vi "Read and Buffer LLP Packets From Host.vi"(0 "channel configuration":T9, 1 "reset":bool, 2 "resources":T1, 12 "ready for output":bool) -> (4 "tagged llp packet":T10, 6 "end of data":bool, 8 "dram status":T19, 10 "output valid":bool)   [LabVIEW 2020, in "GettingStarted_Gen_148X_FPGA.lvlib"]
uses:
  GettingStarted_Gen_148X_FPGA.lvlib
  Common/Types/DRAM Status.ctl
  <instrlib>/FlexRIO/CSI-2/v2/FPGA/Types/Tagged LLP Packet.ctl
  <instrlib>/FlexRIO/CSI-2/v2/FPGA/Types/FPGA LLP Packet Tag.ctl
  <instrlib>/FlexRIO/CSI-2/v2/FPGA/Types/FPGA LLP Packet Timestamp.ctl
  <instrlib>/FlexRIO/CSI-2/v2/FPGA/Types/Timestamp ID.ctl
  <instrlib>/FlexRIO/CSI-2/v2/FPGA/Types/FPGA LLP Packet Size.ctl
  <instrlib>/FlexRIO/CSI-2/v2/FPGA/Types/LLP Packet.ctl
  <instrlib>/FlexRIO/CSI-2/v2/FPGA/Types/LLP Packet Header.ctl
  <instrlib>/FlexRIO/CSI-2/v2/FPGA/Types/LLP Packet Payload.ctl
  <instrlib>/FlexRIO/CSI-2/v2/FPGA/Types/LLP Packet Footer.ctl
  Types/Serial Output Channel Datapath Configuration.ctl
  Types/Serial Output DRAM Resources.ctl
  <instrlib>/_niInstr/Memory/v1/FPGA/DRAM/niInstr Memory DRAM v1 FPGA.lvclass
  <instrlib>/FlexRIO/CSI-2/v2/FPGA/DRAM Manager/Private/DRAM Manager.ctl
  <instrlib>/FlexRIO/CSI-2/v2/FPGA/DRAM Manager/Private/Common/DRAM Manager Registers.ctl
  <instrlib>/FlexRIO/CSI-2/v2/FPGA/DRAM Manager/Private/Common/Handshake Registers.ctl
  <instrlib>/FlexRIO/CSI-2/v2/FPGA/DRAM Manager/Private/Common/DRAM Manager FIFOs.ctl
  <instrlib>/FlexRIO/CSI-2/v2/FPGA/DRAM Manager/Private/Common/Write Data FIFO Ref.ctl
  <instrlib>/FlexRIO/CSI-2/v2/FPGA/DRAM Manager/Private/Common/Read Request Metadata FIFO Ref.ctl
  <instrlib>/FlexRIO/CSI-2/v2/FPGA/DRAM Manager/Private/Common/Read Data FIFO Ref.ctl
  Common/GettingStarted_Common_148X_FPGA.lvlib
  <instrlib>/_niInstr/Basic Elements/v1/FPGA/niInstr Basic Elements v1 FPGA.lvlib
  <instrlib>/FlexRIO/CSI-2/v2/FPGA/NI CSI-2 API FPGA v2.lvlib
  <instrlib>/FlexRIO/CSI-2/v2/FPGA/DRAM Manager/DRAM Manager v2.lvlib
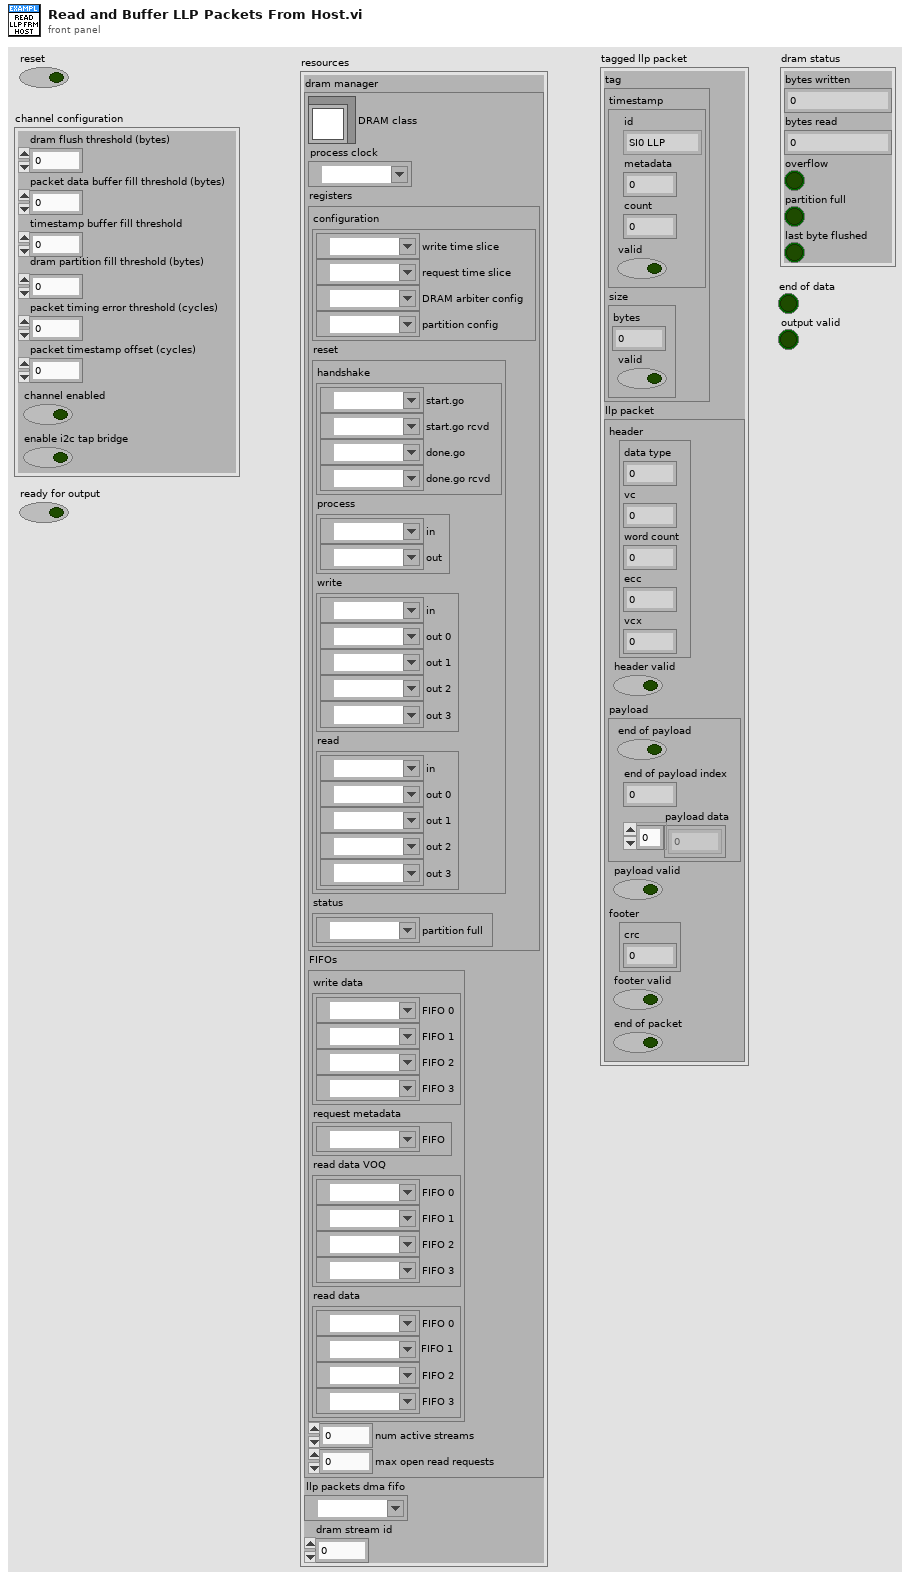
[diagram p1: front panel]
types:
  T1 = typedef "GettingStarted_Gen_148X_FPGA.lvlib/Serial Output DRAM Resources.ctl" = cluster{"dram manager":T2, "llp packets dma fifo":refnum<k21>, "dram stream id":fxp<+,2,2>}
  T2 = typedef "DRAM Manager v2.lvlib/DRAM Manager.ctl" = cluster{"DRAM class":refnum<class "niInstr Memory DRAM v1 FPGA.lvclass">, "process clock":refnum<k21>, "registers":T3, "FIFOs":T5, "num active streams":fxp<+,3,3>, "max open read requests":u16}
  T3 = typedef "DRAM Manager v2.lvlib/DRAM Manager Registers.ctl" = cluster{"configuration":cluster{"write time slice":refnum<k21>, "request time slice":refnum<k21>, "DRAM arbiter config":refnum<k21>, "partition config":refnum<k21>}, "reset":cluster{"handshake":T4, "process":cluster{"in":refnum<k21>, "out":refnum<k21>}, "write":cluster{"in":refnum<k21>, "out 0":refnum<k21>, "out 1":refnum<k21>, "out 2":refnum<k21>, "out 3":refnum<k21>}, "read":cluster{"in":refnum<k21>, "out 0":refnum<k21>, "out 1":refnum<k21>, "out 2":refnum<k21>, "out 3":refnum<k21>}}, "status":cluster{"partition full":refnum<k21>}}
  T4 = typedef "DRAM Manager v2.lvlib/Handshake Registers.ctl" = cluster{"start.go":refnum<k21>, "start.go rcvd":refnum<k21>, "done.go":refnum<k21>, "done.go rcvd":refnum<k21>}
  T5 = typedef "DRAM Manager v2.lvlib/DRAM Manager FIFOs.ctl" = cluster{"write data":cluster{"FIFO 0":T6, "FIFO 1":T6, "FIFO 2":T6, "FIFO 3":T6}, "request metadata":cluster{"FIFO":T7}, "read data VOQ":cluster{"FIFO 0":T8, "FIFO 1":T8, "FIFO 2":T8, "FIFO 3":T8}, "read data":cluster{"FIFO 0":T8, "FIFO 1":T8, "FIFO 2":T8, "FIFO 3":T8}}
  T6 = typedef "DRAM Manager v2.lvlib/Write Data FIFO Ref.ctl" = refnum<k21>
  T7 = typedef "DRAM Manager v2.lvlib/Read Request Metadata FIFO Ref.ctl" = refnum<k21>
  T8 = typedef "DRAM Manager v2.lvlib/Read Data FIFO Ref.ctl" = refnum<k21>
  T9 = typedef "GettingStarted_Gen_148X_FPGA.lvlib/Serial Output Channel Datapath Configuration.ctl" = cluster{"dram flush threshold (bytes)":u64, "packet data buffer fill threshold (bytes)":u64, "timestamp buffer fill threshold":u32, "packet timing error threshold (cycles)":u64, "channel enabled":bool, "dram partition fill threshold (bytes)":u64, "enable i2c tap bridge":bool, "packet timestamp offset (cycles)":i64}
  T10 = typedef "NI CSI-2 API FPGA v2.lvlib/Tagged LLP Packet.ctl" = cluster{"tag":T11, "llp packet":T15}
  T11 = typedef "NI CSI-2 API FPGA v2.lvlib/FPGA LLP Packet Tag.ctl" = cluster{"timestamp":T12, "size":T14}
  T12 = typedef "NI CSI-2 API FPGA v2.lvlib/FPGA LLP Packet Timestamp.ctl" = cluster{"valid":bool, "count":fxp<+,50,50>, "id":T13, "metadata":u8}
  T13 = typedef "NI CSI-2 API FPGA v2.lvlib/Timestamp ID.ctl" = enum8{"SI0 LLP", "SI1 LLP", "SI2 LLP", "SI3 LLP", "SI4 LLP", "SI5 LLP", "SI6 LLP", "SI7 LLP", "SO0 LLP", "SO1 LLP", "SO2 LLP", "SO3 LLP", "SO4 LLP", "SO5 LLP", "SO6 LLP", "SO7 LLP", "Ser0 GPIO Bank", "Ser1 GPIO Bank", "Ser2 GPIO Bank", "Ser3 GPIO Bank", "Ser4 GPIO Bank", "Ser5 GPIO Bank", "Ser6 GPIO Bank", "Ser7 GPIO Bank", "Des0 GPIO Bank", "Des1 GPIO Bank", "Des2 GPIO Bank", "Des3 GPIO Bank", "Des4 GPIO Bank", "Des5 GPIO Bank", "Des6 GPIO Bank", "Des7 GPIO Bank", "User0", "User1", "User2", "User3", "User4", "User5", "User6", "User7", "User8", "User9", "User10", "User11", "User12", "User13", "User14", "User15", "User16", "User17", "User18", "User19", "User20", "User21", "User22", "User23", "User24", "User25", "User26", "User27", "User28", "User29", "User30", "User31"}
  T14 = typedef "NI CSI-2 API FPGA v2.lvlib/FPGA LLP Packet Size.ctl" = cluster{"bytes":fxp<+,17,17>, "valid":bool}
  T15 = typedef "NI CSI-2 API FPGA v2.lvlib/LLP Packet.ctl" = cluster{"header":T16, "header valid":bool, "payload":T17, "payload valid":bool, "footer":T18, "footer valid":bool, "end of packet":bool}
  T16 = typedef "NI CSI-2 API FPGA v2.lvlib/LLP Packet Header.ctl" = cluster{"word count":u16, "ecc":fxp<+,6,6>, "vcx":fxp<+,2,2>, "data type":fxp<+,6,6>, "vc":fxp<+,2,2>}
  T17 = typedef "NI CSI-2 API FPGA v2.lvlib/LLP Packet Payload.ctl" = cluster{"end of payload":bool, "end of payload index":fxp<+,3,3>, "payload data":u8[]}
  T18 = typedef "NI CSI-2 API FPGA v2.lvlib/LLP Packet Footer.ctl" = cluster{"crc":u16}
  T19 = typedef "GettingStarted_Common_148X_FPGA.lvlib/DRAM Status.ctl" = cluster{"bytes written":u64, "bytes read":u64, "overflow":bool, "partition full":bool, "last byte flushed":bool}
  T20 = typedef "niInstr Memory v1 FPGA.lvclass/U256.ctl" = bool[]
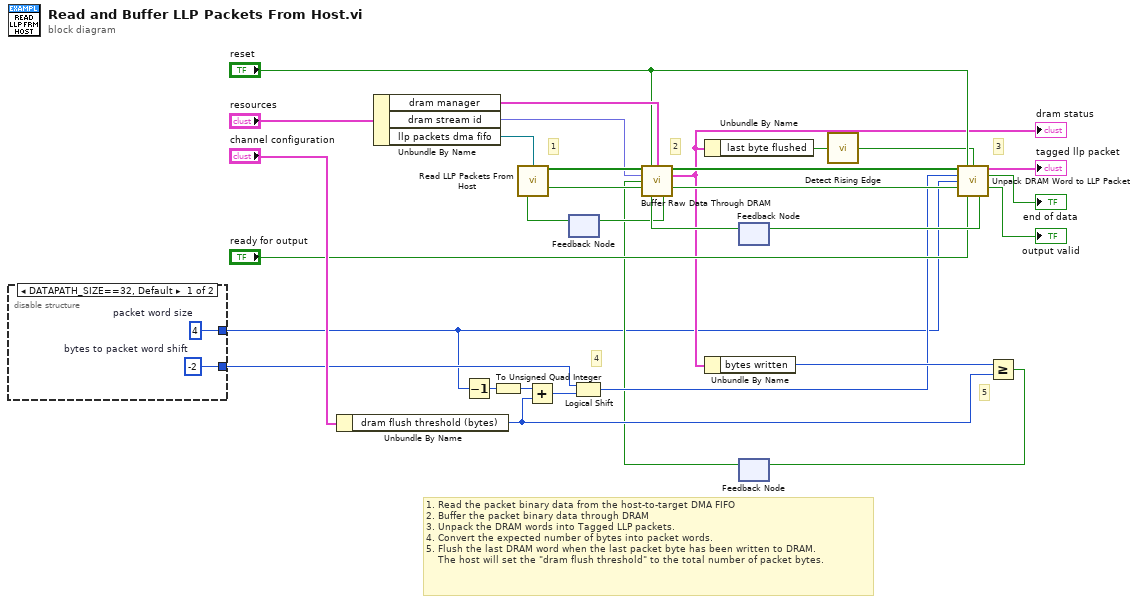
[diagram p0: block diagram]
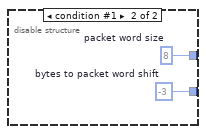
[diagram p2: hidden frame]
diagram:
  # "3"
  # "1. Read the packet binary data from the host-to-target DMA FIFO\n2. Buffer the packet binary data through DRAM\n3. Unpack the DRAM words into Tagged LLP packets.\n4. Convert the expected number of bytes into packet words. \n5. Flush the last DRAM word when the last packet byte has been written to DRAM.\n    The host will set the \"dram flush threshold\" to the total number of packet bytes."
  # "5"
  # "4"
  # "2"
  # "1"
  n1 = disable-structure shown="DATAPATH_SIZE==32, Default" {
    disable-tunnel: [w33 w35] -> w3
    disable-tunnel: [w32 w34] -> w4
    frame condition #0 (active) {
      w32 = i16 -2  # bytes to packet word shift
      w33 = u16 4  # packet word size
    }
    frame condition #1 {
      w34 = i16 -3  # bytes to packet word shift
      w35 = u16 8  # packet word size
    }
  }
  n2 = Unbundle By Name("channel configuration") -> ("dram flush threshold (bytes)"=w13:u64)
  n3 = Unbundle By Name("resources") -> ("dram manager"=w22:T2, "dram stream id"=w21:fxp<+,2,2>, "llp packets dma fifo"=w31:refnum<k21>)
  n4 = Decrement(x=w3) -> (x-1=w2:u16)
  n5 = To Unsigned Quad Integer(1:w2) -> (0:w1:u64)
  n6 = Add(x=w1, y=w13) -> (x+y=w23:u64)
  n7 = feedback #1() -> (w28:bool)  [unwired: 1 in]
  n8 = call "Read LLP Packets From Host.vi"("llp packets dma fifo"=w31, "ready for output"=w28) -> ("dram word"=w24:T20, "output valid"=w26:bool)  [unwired: 12 in]
  n9 = Logical Shift(y=w4, x=w23) -> (x << y=w12:u64)
  n10 = feedback #2() -> (w29:bool)  [unwired: 1 in]
  n11 = feedback #3() -> (w5:bool)  [unwired: 1 in]
  n12 = call "Buffer Raw Data Through DRAM.vi"("dram word in"=w24, "reset"="reset", "dram manager"=w22, "dram stream id"=w21, "flush"=w5, "input valid"=w26, "ready for output"=w29) -> ("dram word out"=w20:T20, "dram status"=w9:T19, "output valid"=w19:bool, "ready for input"=w27:bool)  [unwired: 5 in]
  "dram status" <- w9
  n13 = feedback-in #1(w27) -> ()
  n14 = Unbundle By Name(w9) -> ("last byte flushed"=w8:bool)
  n15 = Unbundle By Name(w9) -> ("bytes written"=w30:u64)
  n16 = call <instrlib>:"Detect Rising Edge.vi"("signal"=w8) -> ("edge detected"=w7:bool)  [unwired: 14 in]
  n17 = call "Unpack DRAM Word to LLP Packet.vi"("dram word"=w20, "reset"="reset", "end of stream"=w7, "expected packet words"=w12, "packet word size"=w3, "input valid"=w19, "ready for output"="ready for output") -> ("tagged llp packet"=→"tagged llp packet":T10, "end of data"=→"end of data":bool, "output valid"=→"output valid":bool, "ready for input"=w18:bool)  [unwired: 5 in]
  n18 = feedback-in #2(w18) -> ()
  n19 = Greater Or Equal?(x=w30, y=w13) -> (x >= y?=w10:bool)
  n20 = feedback-in #3(w10) -> ()
